vi "draw_smiley.vi"() -> ()   [LabVIEW 2024]
panel:
  out "new picture":picture
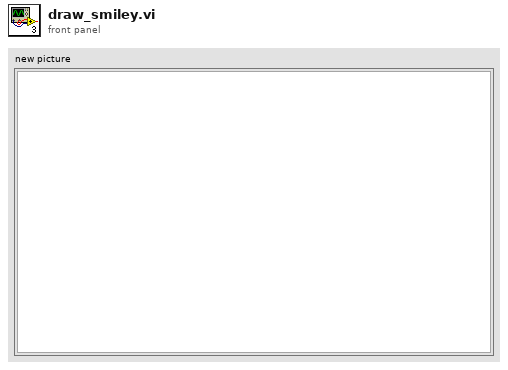
[diagram p1: front panel]
types:
  T1 = cluster{"left":i16, "top":i16, "right":i16, "bottom":i16}
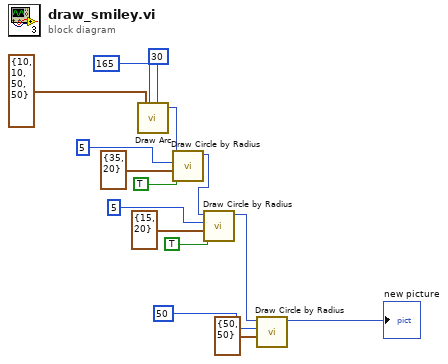
[diagram p0: block diagram]
diagram:
  n1 = call <vilib>:"Draw Arc.vi"("start angle[degrees]"=i16 165, "rect"=T1 {"left"=10, "top"=10, "right"=50, "bottom"=50}, "arc size[degrees]"=i16 30) -> ("new picture"=w4:picture)  [unwired: 6 in]
  n2 = call <vilib>:"Draw Circle by Radius.vi"("fill?(F)"=TRUE, "pixel center"=cluster{"horizontal":i16, "vertical":i16} {"horizontal"=35, "vertical"=20}, "radius"=i16 5, "picture"=w4) -> ("new picture"=w5:picture)  [unwired: 7 in]
  n3 = call <vilib>:"Draw Circle by Radius.vi"("fill?(F)"=TRUE, "pixel center"=cluster{"horizontal":i16, "vertical":i16} {"horizontal"=15, "vertical"=20}, "radius"=i16 5, "picture"=w5) -> ("new picture"=w9:picture)  [unwired: 7 in]
  n4 = call <vilib>:"Draw Circle by Radius.vi"("pixel center"=cluster{"horizontal":i16, "vertical":i16} {"horizontal"=50, "vertical"=50}, "radius"=i16 50, "picture"=w9) -> ("new picture"=→"new picture":picture)  [unwired: 8 in]
